vi "Get Waveform Settings.vi"(8 "error in":errorcluster, 11 "Node Ptr":T1 format="%.0x") -> (0 "error out":errorcluster, 2 "Waveform Settings":T2 {"DataType" items=["Double", "ComplexDouble"]}, 3 "Node Ptr out":T1 format="%.0x")   [LabVIEW 2026]
uses:
  <vilib>/NI VeriStand/Custom Device API/Custom Device Item Ref.ctl
  Types/WaveformSettings.ctl
  NationalInstruments.VeriStand.SystemStorage
  <vilib>/NI VeriStand/Custom Device API/Custom Device API.lvlib
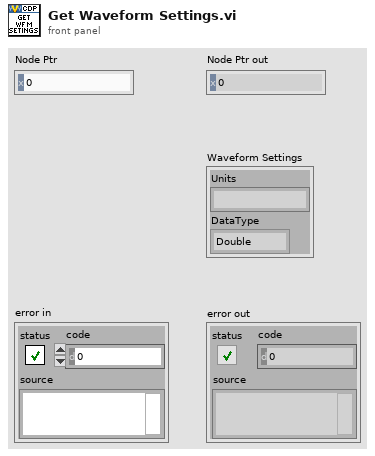
[diagram p1: front panel]
types:
  T1 = typedef "Custom Device API.lvlib/Custom Device Item Ref.ctl" = u64
  T2 = typedef "WaveformSettings.ctl" = cluster{"Units":string, "DataType":i32}
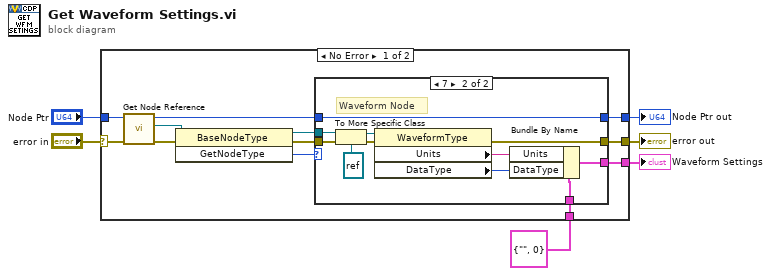
[diagram p0: block diagram]
diagram:
  n1 = case shown="No Error" "error in" {
    selector: "error in" -> [w18 w34]
    tunnel: "Node Ptr" -> [w17 w33]
    tunnel: [w11 w35] -> w5
    tunnel: T2 {"Units"="", "DataType"=0} ("Channel Settings") -> [w10 w35]
    tunnel: [w9 w34] -> w2
    tunnel: [w7 w33] -> w1
    frame No Error {
      n2 = call "Get Node Reference.vi"("error in"=w18, "Node Ptr"=w17) -> ("error out"=w15:errorcluster, "BaseNodeType"=w16:refnum<k24>, "Node Ptr"=w8:T1)  [unwired: 6 in, 1 out]
      n3 = invoke class="BaseNodeType" method="GetNodeType"(reference=w16, error in=w15) -> (reference out=w12:refnum<k24>, error out=w13:errorcluster, "GetNodeType"=w14:i32)  [unwired: 1 in]
      n4 = case shown="7" w14 {
        tunnel: w13 -> [w20 w32]
        tunnel: w12 -> [_ w31]
        tunnel: [w21 w26] -> w11
        tunnel: w10 -> [w21 w25]
        tunnel: [w20 w24] -> w9
        tunnel: [w19 w22] -> w7
        tunnel: w8 -> [w19 w22]
        frame 0, Default {
        }
        frame 7 {
          # "Waveform Node"
          n5 = To More Specific Class(target class=refnum<k24> refnum ("reference"), reference=w31, error in=w32) -> (specific class reference=w29:refnum<k24>, error out=w28:errorcluster)
          n6 = property class="WaveformType"(reference=w29, error in=w28) -> (error out=w24:errorcluster, "Units"=w27:string, "DataType"=w23:i32)  [unwired: 1 out]
          n7 = Bundle By Name(cluster=w25, "Units"=w27, "DataType"=w23) -> (w26:T2)
        }
      }
    }
    frame Error {
    }
  }
  "Waveform Settings" <- w5
  "error out" <- w2
  "Node Ptr out" <- w1
